vi "X Listbox Facade - Challenge.vi"(0 "Data In":T4, 2 "Display State In":T2, 3 "Container State":T3) -> (6 "Data Out":T4, 7 "Display State Out":T2, 8 "Action":T1)   [LabVIEW 2009]
doc: "This VI is missing some links but simple shows the solution to one of the challenges.\n\nAAL 9/09"
uses:
  <vilib>/_xctls/Action.ctl
  <vilib>/_xctls/XControlSupport.lvlib
  <vilib>/_xctls/Container State.ctl
  X Listbox Data.ctl
  X Listbox State.ctl
panel:
  in  "Listbox":i32(listbox)
  in  "True Boolean":bool=TRUE
  in  "False Boolean":bool
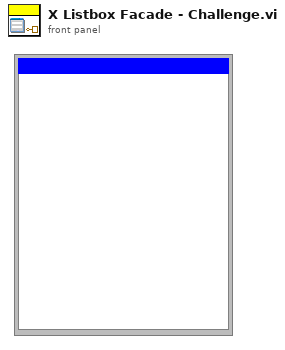
[diagram p1: front panel]
types:
  T1 = typedef "XControlSupport.lvlib/Action.ctl" = cluster{"Data Changed?":bool, "State Changed?":bool, "Action Name":string}
  T2 = typedef "X Listbox.xctl/X Listbox State.ctl" = cluster{"# Items":i32, "Names":string[]}
  T3 = typedef "XControlSupport.lvlib/Container State.ctl" = cluster{"Indicator?":bool, "Run Mode?":bool, " Refnum":refnum<vi>}
  T4 = typedef "X Listbox.xctl/X Listbox Data.ctl" = string
  T5 = typedef "LVPoint32TypeDef.ctl" = cluster{"Horizontal":i32, "Vertical":i32}
  T6 = typedef "imagedata.ctl" = cluster{"image type":i32, "image depth":i32, "image":u8[], "mask":u8[], "colors":u32[], "Rectangle":cluster{"left":i16, "top":i16, "right":i16, "bottom":i16}}
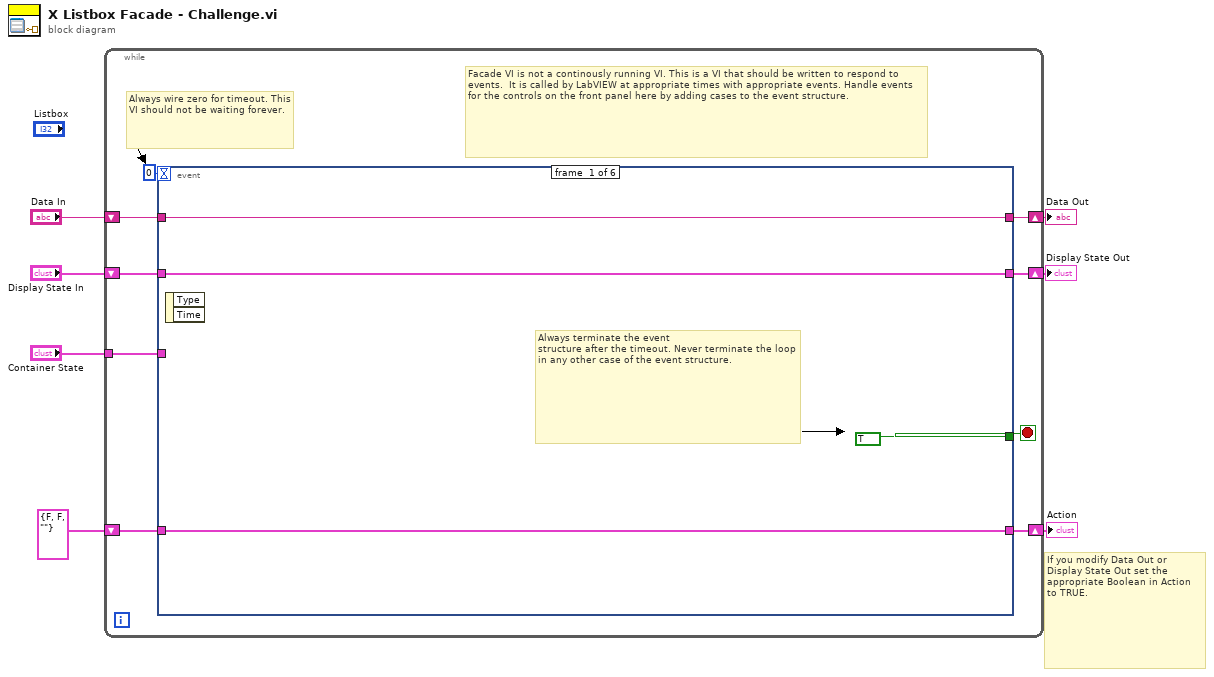
[diagram p0: block diagram]
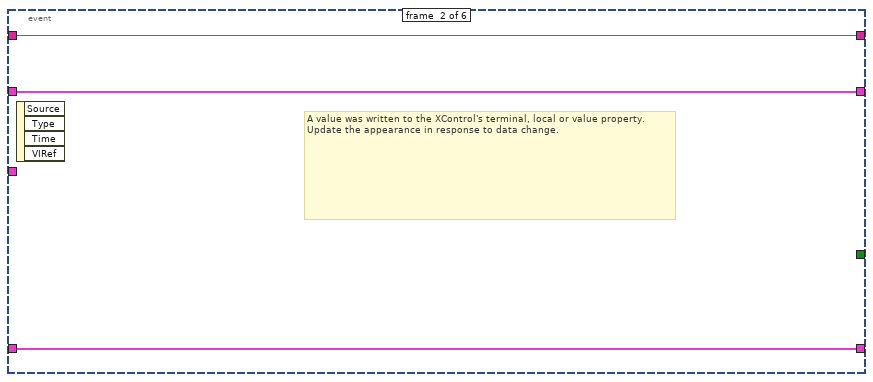
[diagram p2: hidden frame]
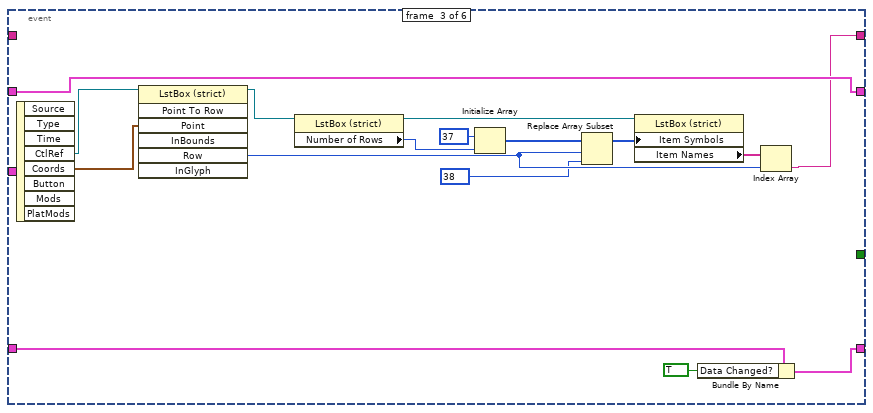
[diagram p3: hidden frame]
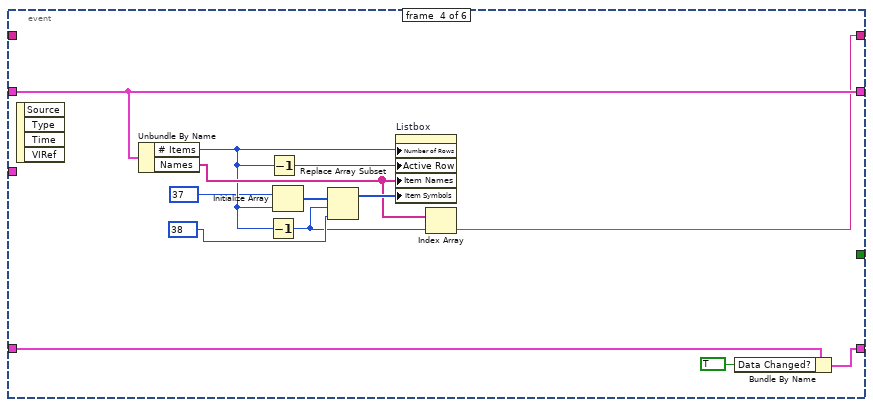
[diagram p4: hidden frame]
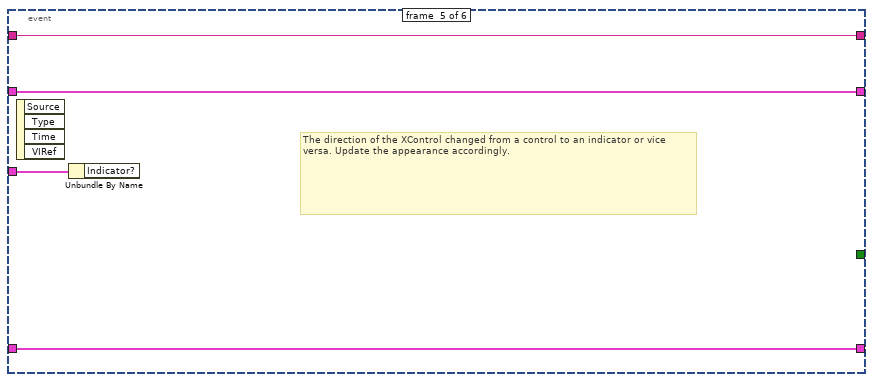
[diagram p5: hidden frame]
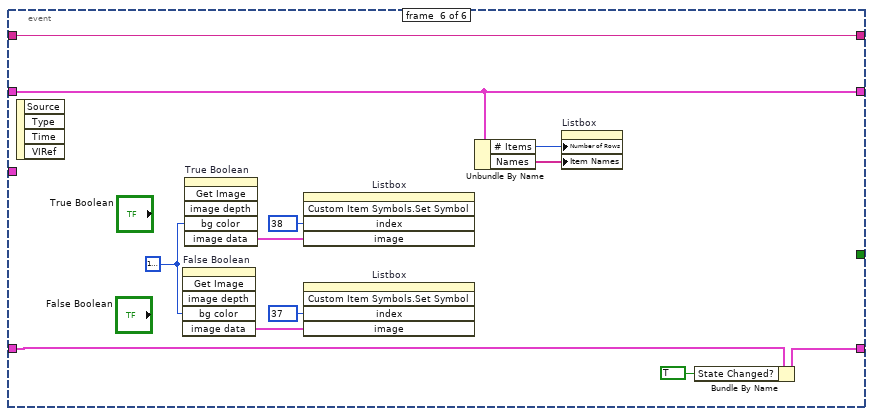
[diagram p6: hidden frame]
diagram:
  # "If you modify Data Out or\nDisplay State Out set the\nappropriate Boolean in Action\nto TRUE."
  n1 = while {
    shift-right: [w15] -> w4
    shift-left: "Display State In" -> [w16]
    tunnel: "Container State" -> [w12]
    shift-right: [w10] -> w7
    shift-left: "Data In" -> [w11]
    shift-right: [w8] -> w2
    shift-left: T1 {"Data Changed?"=FALSE, "State Changed?"=FALSE, "Action Name"=""} ("Action") -> [w9]
    stop <- w14 stop-if-true
    # "Facade VI is not a continously running VI. This is a VI that should be written to respond to events.  It is called by LabVIEW at appropriate times with appropriate events. Handle events for the controls on the front panel here by adding cases to the event structure."
    # "Always wire zero for timeout. This\nVI should not be waiting forever."
    n2 = event shown="[5] Exec State Change" {
      selector: _ -> [_ _ _ _ _ _]
      dyn-events: _ -> [_ _ _ _ _ _]
      timeout: 0 -> [_ _ _ _ _ _]
      tunnel: w16 -> [w18 w22 w35 w52 w55 w59]
      tunnel: [w18 w22 w35 w52 w55 w59] -> w15
      tunnel: [TRUE _ _ _ _ _] -> w14
      tunnel: w12 -> [_ _ _ _ w56 _]
      tunnel: w11 -> [w17 w23 _ _ w54 w68]
      tunnel: [w17 w23 w34 w42 w54 w68] -> w10
      tunnel: [w19 w21 w32 w46 w53 w60] -> w8
      tunnel: w9 -> [w19 w21 w33 w47 w53 w67]
      event #0 {
        # "Always terminate the event\nstructure after the timeout. Never terminate the loop in any other case of the event structure."
        n3 = event-data() -> ()  [unwired: 3 out]
      }
      event #1 {
        # "A value was written to the XControl's terminal, local or value property.\nUpdate the appearance in response to data change."
        n4 = event-data() -> ()  [unwired: 5 out]
      }
      event #2 {
        n5 = event-data() -> ("CtlRef"=w39:refnum<vi>, "Coords"=w36:T5)  [unwired: 7 out]
        n6 = invoke class="LstBox (strict)" method="Point To Row"(reference=w39, "Point"=w36) -> (reference out=w38:refnum<vi>, "Row"=w37:i32)  [unwired: 5 in, 5 out]
        n7 = property class="LstBox (strict)"(reference=w38) -> (reference out=w30:refnum<vi>, "Number of Rows"=w26:u32)  [unwired: 1 in, 1 out]
        n8 = Initialize Array(37, w26) -> (w24:i32[])
        n9 = Replace Array Subset(array=w24, new element=38, index=w37) -> (w29:i32[])
        n10 = property class="LstBox (strict)"(reference=w30, "Item Symbols"=w29) -> ("Item Names"=w28:string[])  [unwired: 1 in, 2 out]
        n11 = Bundle By Name(cluster=w33, "Data Changed?"=TRUE) -> (w32:T1)
        n12 = Index Array(array=w28, index=w37) -> (element=w34:string)
      }
      event #3 {
        n13 = event-data() -> ()  [unwired: 5 out]
        n14 = Unbundle By Name(w52) -> ("# Items"=w41:i32, "Names"=w44:string[])
        n15 = Decrement(x=w41) -> (x-1=w43:i32)
        n16 = Decrement(x=w41) -> (x-1=w51:i32)
        n17 = Initialize Array(37, w41) -> (w50:i32[])
        n18 = Replace Array Subset(array=w50, new element=38, index=w43) -> (w48:i32[])
        n19 = property on="Listbox" class="LstBox (strict)"("Number of Rows"=w41, "Active Row"=w51, "Item Names"=w44, "Item Symbols"=w48) -> ()  [unwired: 2 in, 2 out]
        n20 = Index Array(array=w44, index=w43) -> (element=w42:string)
        n21 = Bundle By Name(cluster=w47, "Data Changed?"=TRUE) -> (w46:T1)
      }
      event #4 {
        # "The direction of the XControl changed from a control to an indicator or vice versa. Update the appearance accordingly."
        n22 = event-data() -> ()  [unwired: 5 out]
        n23 = Unbundle By Name(w56) -> ()  [unwired: 1 out]
      }
      event #5 {
        w64 = u32 16777226
        n24 = event-data() -> ()  [unwired: 5 out]
        n25 = invoke on="False Boolean" class="Bool (strict)" method="Get Image"("bg color"=w64) -> ("image data"=w63:T6)  [unwired: 5 in, 5 out]
        n26 = invoke on="True Boolean" class="Bool (strict)" method="Get Image"("bg color"=w64) -> ("image data"=w62:T6)  [unwired: 5 in, 5 out]
        n27 = invoke on="Listbox" class="LstBox (strict)" method="Custom Item Symbols.Set Symbol"("index"=38, "image"=w62) -> ()  [unwired: 3 in, 5 out]
        n28 = invoke on="Listbox" class="LstBox (strict)" method="Custom Item Symbols.Set Symbol"("index"=37, "image"=w63) -> ()  [unwired: 3 in, 5 out]
        n29 = Unbundle By Name(w59) -> ("# Items"=w58:i32, "Names"=w57:string[])
        n30 = property on="Listbox" class="LstBox (strict)"("Number of Rows"=w58, "Item Names"=w57) -> ()  [unwired: 2 in, 2 out]
        n31 = Bundle By Name(cluster=w67, "State Changed?"=TRUE) -> (w60:T1)
      }
    }
  }
  "Display State Out" <- w4
  "Data Out" <- w7
  "Action" <- w2
